vi "FTW-CodeGen-OnFontOrLocaleChange.vi"(0 "State In":T1, 5 "XRef":refnum<vi>) -> (4 "State Out":T1, 6 "Reply":string[](array[string]))   [LabVIEW 2015, in "FTW-Actor-Ask.xnode"]
uses:
  FTW-Actor-Ask.xnode
  FTW-CodeGen-State.ctl
  src/reflection/FTW-Reflection-Types.ctl
  FTW-CodeGen-XNodeReplyType.ctl
panel:
  # "Inputs"
  # "Outputs"
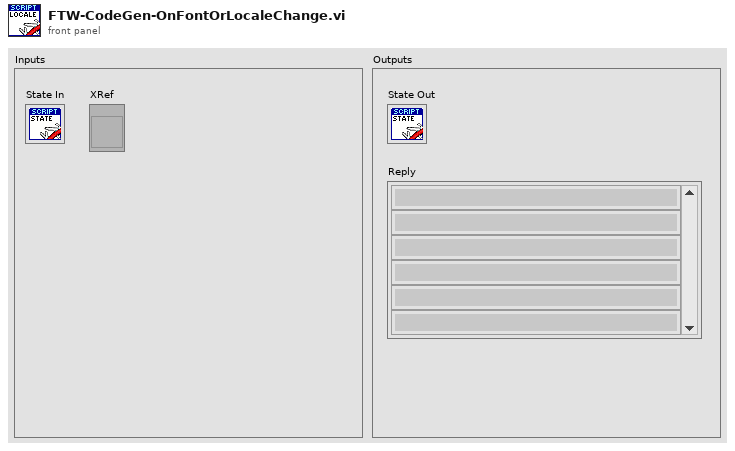
[diagram p1: front panel]
types:
  T1 = typedef "FTW-Actor-Ask.xnode/FTW-CodeGen-State.ctl" = cluster{"Request Type":T2, "Response Type":T2}
  T2 = typedef "FTW-Reflection-Types.ctl" = enum16{"Unknown", "Void", "Array", "Cluster", "LVObject", "Boolean", "I8", "I16", "I32", "I64", "U8", "U16", "U32", "U64", "SGL", "DBL", "EXT", "CSG", "CDB", "CXT", "FXP", "EnumU8", "EnumU16", "EnumU32", "EnumU64", "SGLwithUnit", "DBLwithUnit", "EXTwithUnit", "CSGwithUnit", "CDBwithUnit", "CXTwithUnit", "String", "Path", "Picture", "Tag", "LVVariant", "Timestamp", "WaveformI8", "WaveformI16", "WaveformI32", "WaveformI64", "WaveformU8", "WaveformU16", "WaveformU32", "WaveformU64", "WaveformSGL", "WaveformDBL", "WaveformEXT", "WaveformCSG", "WaveformCDB", "WaveformCXT", "WaveformDigital", "WaveformUnknownType", "DigitalData", "DynamicData", "ExternalData", "FileByteStream", "TDMStream", "dotNET", "ActiveX", "VIServerReference", "VIReference", "ApplicationInstance", "Menu", "ConnectionDataSocket", "ConnectionVISA", "ConnectionBluetooth", "ConnectionIrDA", "ConnectionTCP", "ConnectionUDP", "ConnectionHTTPClient", "ConnectionFTP", "Occurrence", "Notifier", "Queue", "Rendezvous", "Semaphore", "RTFIFO", "EventPublisher", "EventRegistration", "EventCallback", "DataValueReference", "GenericClass", "GenericClassTag", "GenericClassDeepCopy", "GenericClassFlattened", "GenericClassTagFlattened", "GenericReferenceType", "WindowsRegistry", "OverloadedDatalogRef", "ReferenceUnknownType", "ByteArray", "ConPaneInterface", "FTWObject"}
  T3 = typedef "FTW-CodeGen-XNodeReplyType.ctl" = enum16{"UpdateState", "AdaptToInputs", "AdaptAndAugment", "CosmeticUpdate", "NoReply"}
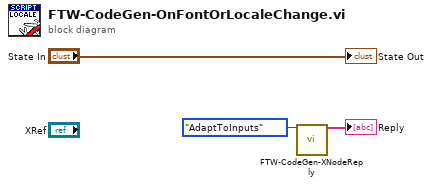
[diagram p0: block diagram]
diagram:
  n1 = call "FTW-CodeGen-XNodeReply.vi"("XNode Reply Type"=FTW-CodeGen-XNodeReplyType."AdaptToInputs") -> ("Reply"=→"Reply":string[])  [unwired: 14 in]
  "State Out" <- "State In"
